vi "API_DB.GetLocationForReticleID.vi"(0 "Database in":refnum<class "Database.lvclass">, 1 "Wait (F)":bool, 5 "Table":string, 7 "InventoryRecord.ReticleID":string, 11 "error in (no error)":errorcluster, 12 "Timeout (ms)":u32) -> (4 "Database out":refnum<class "Database.lvclass">, 6 "Slot":string, 15 "error out":errorcluster)   [LabVIEW 2020, in "Database.lvclass"]
doc: "Developed by Kevin Thompson\nkevin@thompsonengineering.net\n\nCopyright 2018\nThompson Engineering, LLC"
uses:
  Database.lvclass
  DataTypes/AsynCmd_Temp01--enum.ctl
  DataTypes/GenericQuery--Cluster.ctl
  DataTypes/SQLQuery--Enum.ctl
  DataTypes/InventoryRecord--Cluster.ctl
  DataTypes/Module--Cluster.ctl
  DataTypes/LocationStatus--Enum.ctl
  Database.lvclass/Database.ctl
  DataTypes/Stocker--Enum.ctl
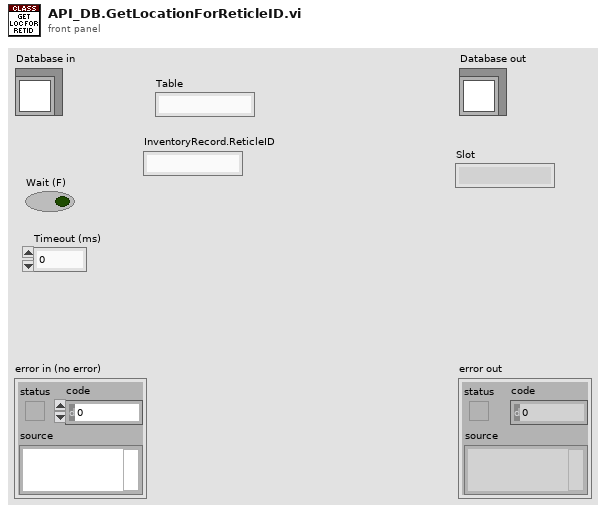
[diagram p1: front panel]
types:
  T1 = typedef "SQLQuery--Enum.ctl" = enum16{"GetInventoryRecordFromDB", "GetReticleInfoFromDB", "GetLocationStatusFromDB", "UpdateInventoryRecord", "UpdateLocationStatus", "UpdateReticleLocationStatus", "AddReticleInDB", "RemoveReticleAtLocation", "RemoveReticleUsingReticleID", "GetLocationForReticleID", "GetAllLocations", "GetAllEmptyLocations", "GetAllLocationsInStocker", "GetAllFullLocations", "GetAllFullLocationsInStocker", "GetAllDisabledLocations", "GetAllDisabledLocationsInStocker", "FindFirstSlot"}
  T2 = typedef "GenericQuery--Cluster.ctl" = cluster{"Query":T1, "Table":string, "InventoryRecord":T3}
  T3 = typedef "InventoryRecord--Cluster.ctl" = cluster{"ReticleID":string, "Stocker":T4, "Location":T5, "LocationStatus":T6, "EquipmentID":string, "LocationID":string}
  T4 = typedef "Stocker--Enum.ctl" = u16
  T5 = typedef "Module--Cluster.ctl" = cluster{"Module":u16, "Row":u16, "Column":u16}
  T6 = typedef "LocationStatus--Enum.ctl" = enum16{"Disabled/Unusable", "Full", "Empty"}
  T7 = typedef "Database.lvclass/AsynCmd_Temp01--enum.ctl" = enum16{"DB.DeleteRecord", "DB.UpdateRecord", "DB.InsertRecord", "DB.SelectRecord", "DB.ExecuteSQLCommand", "DB.FindFirstSlot", "DB.GenericSQLQuery"}
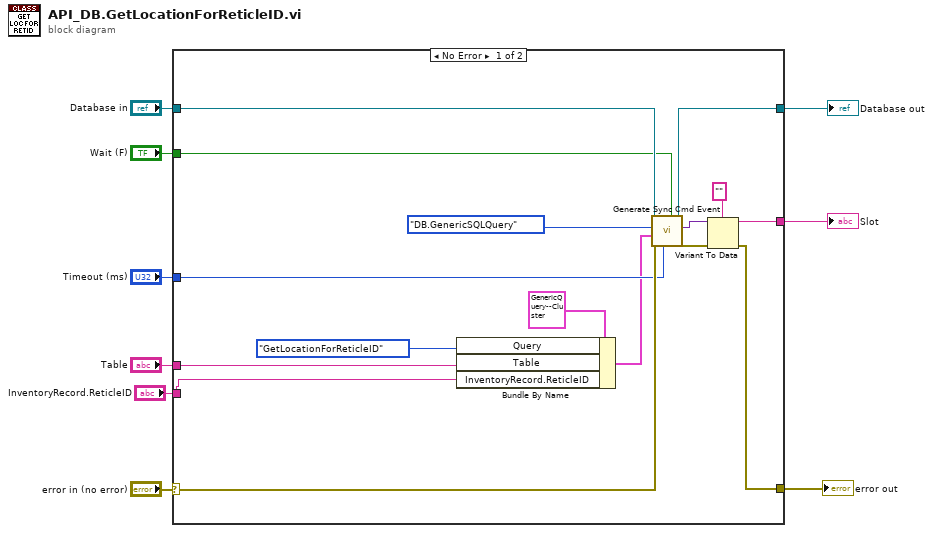
[diagram p0: block diagram]
diagram:
  n1 = case shown="No Error" "error in (no error)" {
    selector: "error in (no error)" -> [w23 w27]
    tunnel: [w18 w27] -> w8
    tunnel: [w24 w26] -> w6
    tunnel: "Database in" -> [w25 w26]
    tunnel: [w20 _] -> w3
    tunnel: "Wait (F)" -> [w17 _]
    tunnel: "Timeout (ms)" -> [w16 _]
    tunnel: "Table" -> [w11 _]
    tunnel: "InventoryRecord.ReticleID" -> [w10 _]
    frame No Error {
      n2 = Bundle By Name(cluster=T2 {"Query"=enum."GetInventoryRecordFromDB", "Table"="", "InventoryRecord"={"ReticleID"="", "Stocker"=0, "Location"={"Module"=0, "Row"=0, "Column"=0}, "LocationStatus"=enum."Disabled/Unusable", "EquipmentID"="", "LocationID"=""}}, "Query"=SQLQuery--Enum."GetLocationForReticleID", "Table"=w11, "InventoryRecord.ReticleID"=w10) -> (w12:T2)
      n3 = call "Generate Sync Cmd Event.vi"("Wait (F)"=w17, "Timeout (ms)"=w16, "error in (no error)"=w23, "vData"=w12, "AsyncCmd"=AsynCmd_Temp01--enum."DB.GenericSQLQuery", "Database in"=w25) -> ("error out"=w19:errorcluster, "Return Value"=w21:variant, "Database out"=w24:refnum<class "Database.lvclass">)  [unwired: 3 in]
      n4 = Variant To Data(error in=w19, type="", Variant=w21) -> (data=w20:string, error out=w18:errorcluster)
    }
    frame Error {
    }
  }
  "error out" <- w8
  "Database out" <- w6
  "Slot" <- w3
